vi "Sweep.vi"() -> ()   [LabVIEW 2020]
uses:
  <instrlib>/Keithley 2600 Series/Public/Configure/Source/Configure Source (Range).vi
  <instrlib>/Keithley 2600 Series/Public/Configure/Source/Configure Source (Level).vi
  <instrlib>/Keithley 2600 Series/Public/Configure/Source/Configure Source (Limit).vi
  <instrlib>/Keithley 2600 Series/Public/Data/Read Measurement (Current).vi
  <instrlib>/Keithley 2600 Series/Public/Data/Read Current (Linear Voltage Sweep).vi
  <instrlib>/Keithley 2600 Series/Keithley 2600 Series.lvlib
panel:
  in  "Pulse Stop Level (1 V)":dbl=1.0
  in  "Pulse Start Level (0 V)":dbl
  in  "Sweep Points (10)":i32=10
  in  "Delay Time (0.01 S)":dbl=0.01
  out "Current (A)":dbl[](array[numeric])
  out "Current Buffer Data (A)":dbl[](array[numeric])
  in  "Measurement Count (10)":i32=10
  in  "Current Limit (0.1 A)":dbl=0.1
  in  "Voltage Level (1 V)":dbl=1.0
  in  "SMU Channel (0: Channel A)":i32(ring) items=["Channel A", "Channel B"]
  in  "VISA resource name":refnum<visa-resource-name>
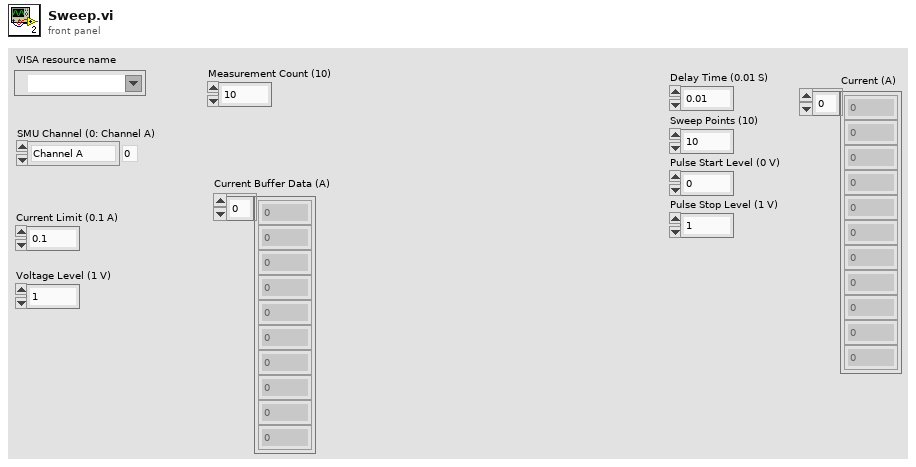
[diagram p1: front panel]
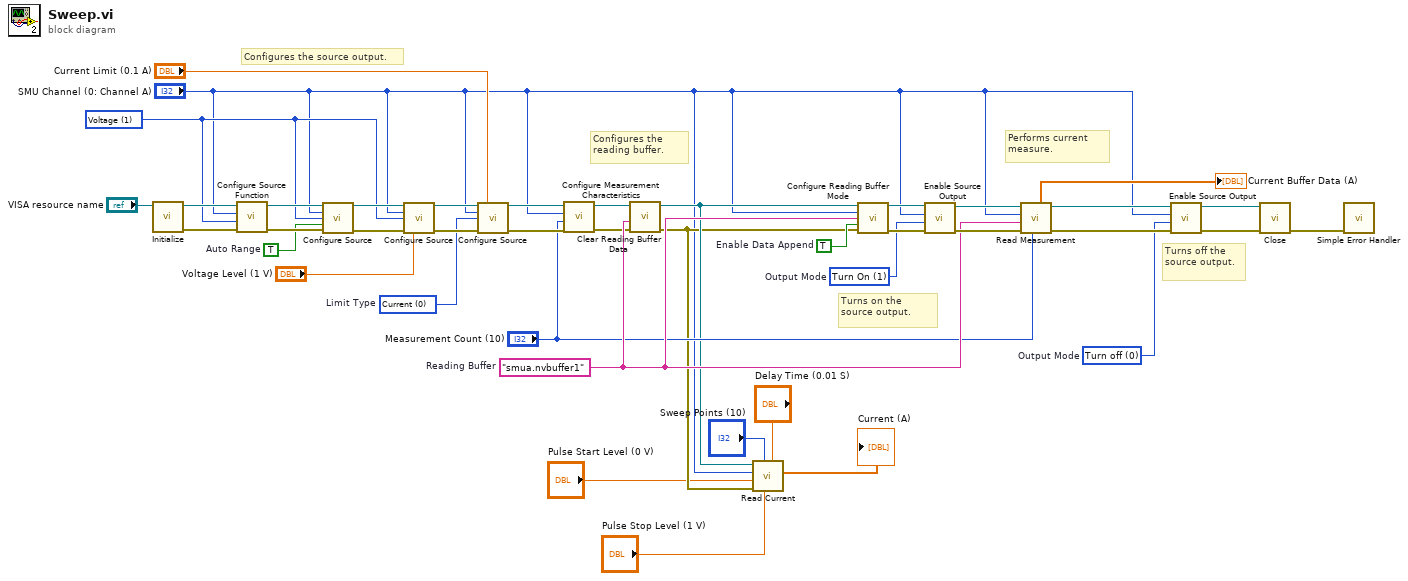
[diagram p0: block diagram]
diagram:
  w30 = 1 items=["Voltage"=1] ("Source Function (1: Voltage)")
  w9 = 0 items=["Current", "Voltage", "Power"]  # Limit Type
  w19 = 0 items=["Turn off", "Turn On", "High-Z"]  # Output Mode
  w25 = 1 items=["Turn off", "Turn On", "High-Z"]  # Output Mode
  w28 = TRUE  # Enable Data Append
  w22 = "smua.nvbuffer1"  # Reading Buffer
  w34 = TRUE  # Auto Range
  # "Turns on the source output."
  # "Configures the reading buffer."
  # "Configures the source output."
  # "Performs current measure."
  # "Turns off the source output."
  n1 = call <instrlib>:"Initialize.vi"("VISA resource name"="VISA resource name") -> ("error out"=w39:errorcluster, "VISA resource name out"=w40:refnum<visa-resource-name>)  [unwired: 9 in]
  n2 = call <instrlib>:"Configure Source Function.vi"("error in (no error)"=w39, "Source Function (1: Voltage)"=w30, "Source Measure Unit Channel (0: Channel A)"="SMU Channel (0: Channel A)", "VISA resource name"=w40) -> ("error out"=w37:errorcluster, "VISA resource name out"=w38:refnum<visa-resource-name>)  [unwired: 6 in]
  n3 = call-poly <instrlib>:"Configure Source.vi"("VISA resource name"=w38, "Source Measure Unit Channel (0: Channel A)"="SMU Channel (0: Channel A)", "Range Type (1: Voltage)"=w30, "Auto Range (T: Enable)"=w34, "error in (no error)"=w37) -> ("VISA resource name out"=w36:refnum<visa-resource-name>, "error out"=w35:errorcluster)  [unwired: 9 in]
  n4 = call-poly <instrlib>:"Configure Source.vi"("VISA resource name"=w36, "Source Measure Unit Channel (0: Channel A)"="SMU Channel (0: Channel A)", "Level Type (1: Voltage)"=w30, "error in (no error)"=w35, "Voltage Level (0 V)"="Voltage Level (1 V)") -> ("VISA resource name out"=w32:refnum<visa-resource-name>, "error out"=w31:errorcluster)  [unwired: 9 in]
  n5 = call-poly <instrlib>:"Configure Source.vi"("VISA resource name"=w32, "Current Limit (0.1 A)"="Current Limit (0.1 A)", "Source Measure Unit Channel (0: Channel A)"="SMU Channel (0: Channel A)", "Limit Type (1: Voltage)"=w9, "error in (no error)"=w31) -> ("VISA resource name out"=w18:refnum<visa-resource-name>, "error out"=w17:errorcluster)  [unwired: 9 in]
  n6 = call <instrlib>:"Configure Measurement Characteristics.vi"("error in (no error)"=w17, "Measurement Count (1)"="Measurement Count (10)", "Source Measure Unit Channel (0: Channel A)"="SMU Channel (0: Channel A)", "VISA resource name"=w18) -> ("error out"=w15:errorcluster, "VISA resource name out"=w16:refnum<visa-resource-name>)  [unwired: 6 in]
  n7 = call <instrlib>:"Clear Reading Buffer Data.vi"("error in (no error)"=w15, "Reading Buffer (smua.nvbuffer1)"=w22, "VISA resource name"=w16) -> ("error out"=w7:errorcluster, "VISA resource name out"=w8:refnum<visa-resource-name>)  [unwired: 7 in]
  n8 = call-poly <instrlib>:"Read Current.vi"("Delay Time (0.01 S)"="Delay Time (0.01 S)", "Pulse Stop Level (1 V)"="Pulse Stop Level (1 V)", "Sweep Points (10)"="Sweep Points (10)", "error in (no error)"=w7, "Pulse Start Level (0 V)"="Pulse Start Level (0 V)", "Source Measure Unit Channel (0: Channel A)"="SMU Channel (0: Channel A)", "VISA resource name"=w8) -> ("Current (A)"=→"Current (A)":dbl[])  [unwired: 2 in, 2 out]
  n9 = call <instrlib>:"Configure Reading Buffer Mode.vi"("VISA resource name"=w8, "Source Measure Unit Channel (0: Channel A)"="SMU Channel (0: Channel A)", "Reading Buffer (smua.nvbuffer1)"=w22, "Enable Data Append (F: Disable)"=w28, "error in (no error)"=w7) -> ("VISA resource name out"=w27:refnum<visa-resource-name>, "error out"=w26:errorcluster)  [unwired: 9 in]
  n10 = call <instrlib>:"Enable Source Output.vi"("error in (no error)"=w26, "Output Mode (0: Turn off)"=w25, "Source Measure Unit Channel (0: Channel A)"="SMU Channel (0: Channel A)", "VISA resource name"=w27) -> ("error out"=w23:errorcluster, "VISA resource name out"=w24:refnum<visa-resource-name>)  [unwired: 6 in]
  n11 = call-poly <instrlib>:"Read Measurement.vi"("Wait Time (10 S)"="Measurement Count (10)", "error in (no error)"=w23, "Current Buffer (smua.nvbuffer1)"=w22, "Source Measure Unit Channel (0: Channel A)"="SMU Channel (0: Channel A)", "VISA resource name"=w24) -> ("error out"=w20:errorcluster, "VISA resource name out"=w21:refnum<visa-resource-name>, "Current Buffer Data (A)"=→"Current Buffer Data (A)":dbl[])  [unwired: 3 in, 1 out]
  n12 = call <instrlib>:"Enable Source Output.vi"("error in (no error)"=w20, "Output Mode (0: Turn off)"=w19, "Source Measure Unit Channel (0: Channel A)"="SMU Channel (0: Channel A)", "VISA resource name"=w21) -> ("error out"=w11:errorcluster, "VISA resource name out"=w12:refnum<visa-resource-name>)  [unwired: 6 in]
  n13 = call <instrlib>:"Close.vi"("error in (no error)"=w11, "VISA resource name"=w12) -> ("error out"=w10:errorcluster)  [unwired: 9 in]
  n14 = call <vilib>:"Simple Error Handler.vi"("error in (no error)"=w10) -> ()  [unwired: 4 in, 5 out]
